vi "Main.vi"() -> ()   [LabVIEW 2018]
uses:
  TicTacToeControl.ctl
panel:
  out "array":string[](array[string])
  in  "stop":bool
  out "Display":string
  in  "Board":T1
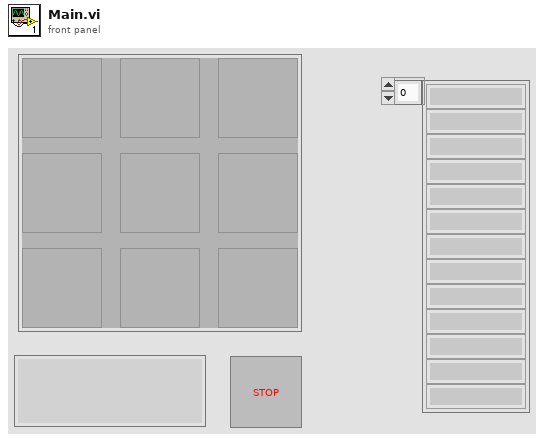
[diagram p1: front panel]
types:
  T1 = cluster{"OK Button":bool, "OK Button 2":bool, "OK Button 3":bool, "OK Button 4":bool, "OK Button 5":bool, "OK Button 6":bool, "OK Button 7":bool, "OK Button 8":bool, "OK Button 9":bool}
  T2 = typedef "TicTacToeControl.ctl" = enum16{"Initialize", "GetUserInput", "GetComputerMove", "SetControlValue", "Initialize Control References", "Wait for Event", "Quit", "Play Again ?", "Check result ?"}
  T3 = cluster{"Controls[]":refnum<vi>[], "selection index":i32, "user symbol":string, "computer symbol":string}
  T4 = typedef "gameStatus.ctl" = enum16{"player won", "computer won", "draw", "no result"}
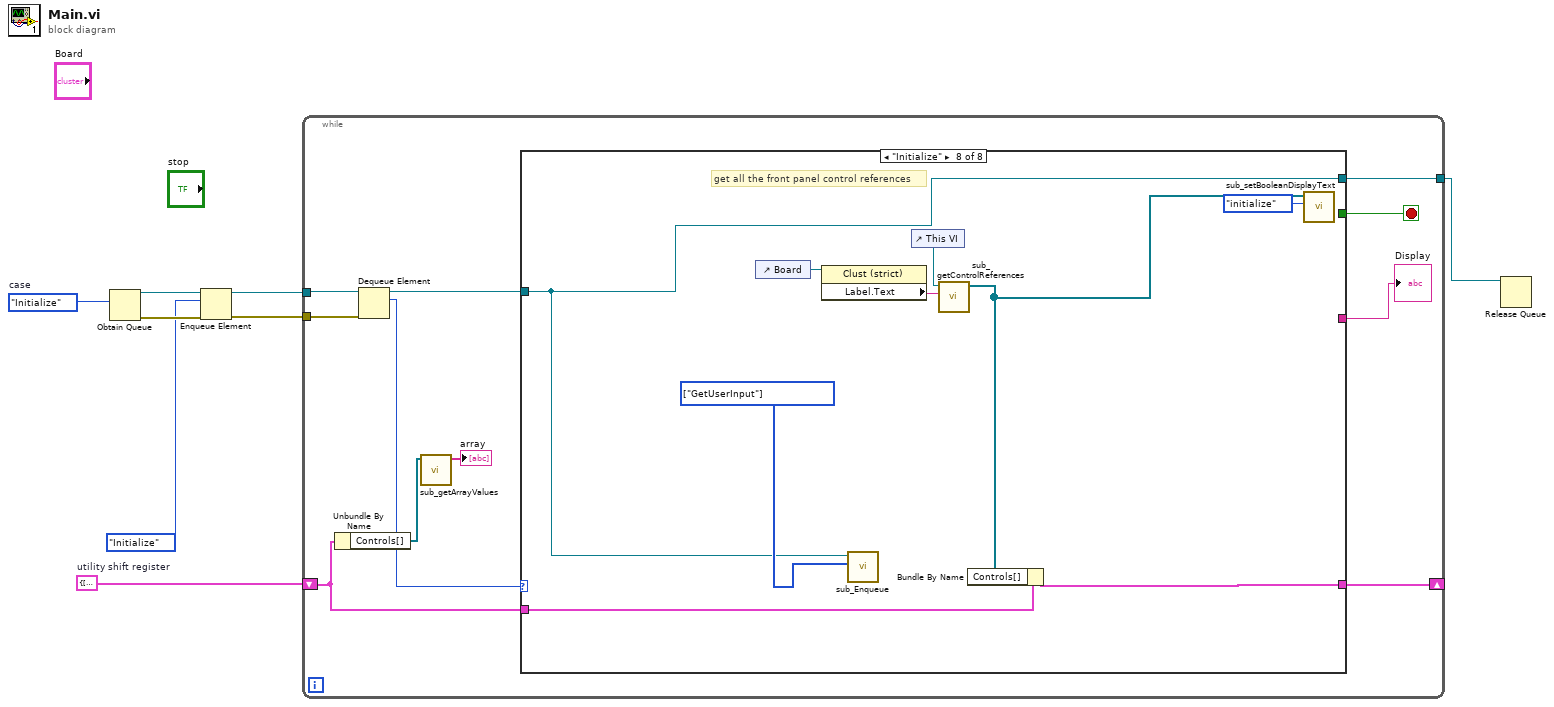
[diagram p0: block diagram]
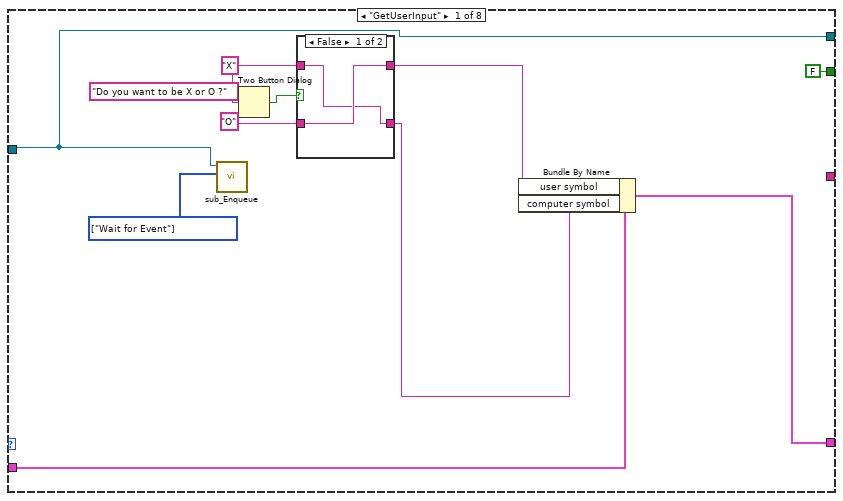
[diagram p2: hidden frame]
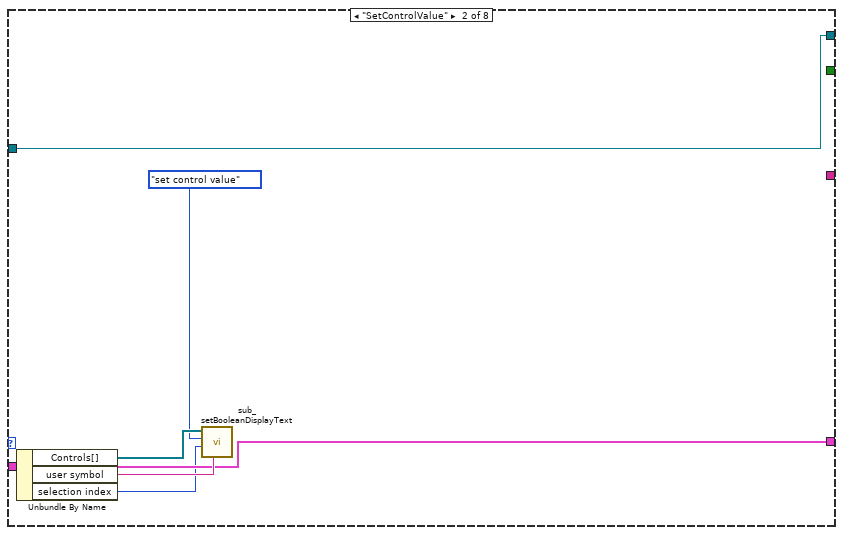
[diagram p4: hidden frame]
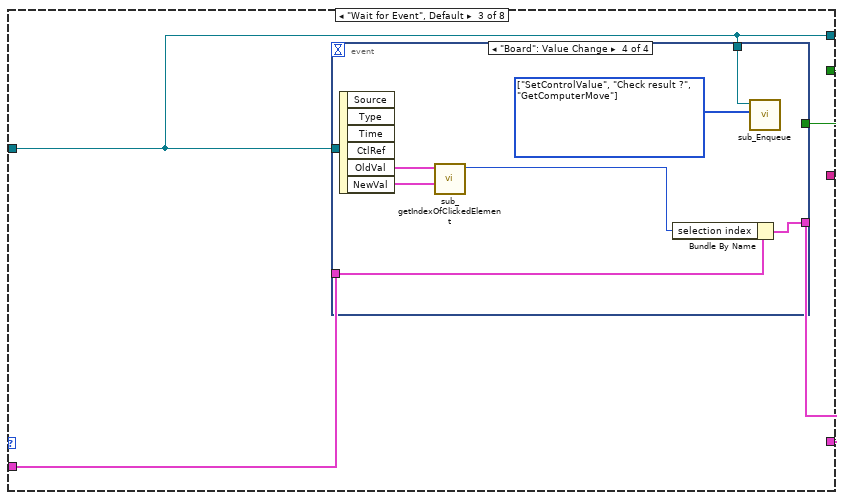
[diagram p5: hidden frame]
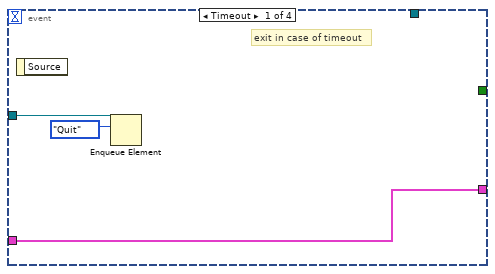
[diagram p6: hidden frame]
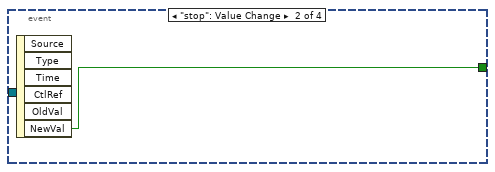
[diagram p7: hidden frame]
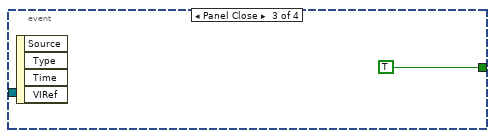
[diagram p8: hidden frame]
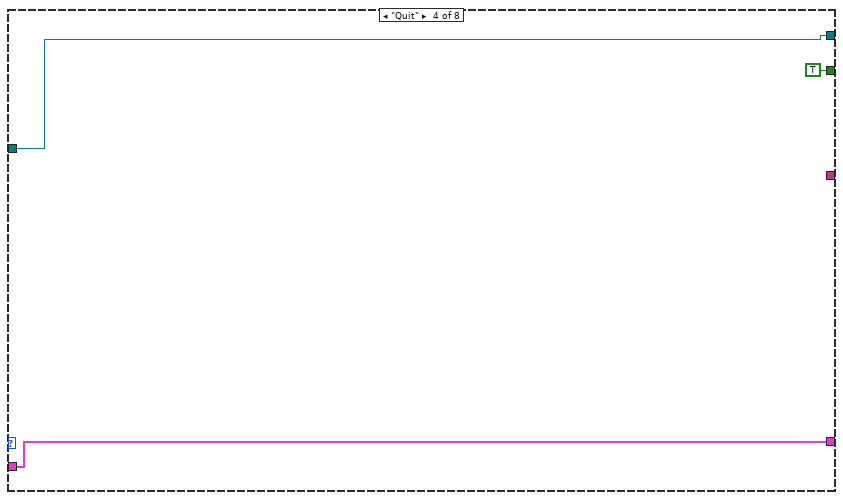
[diagram p9: hidden frame]
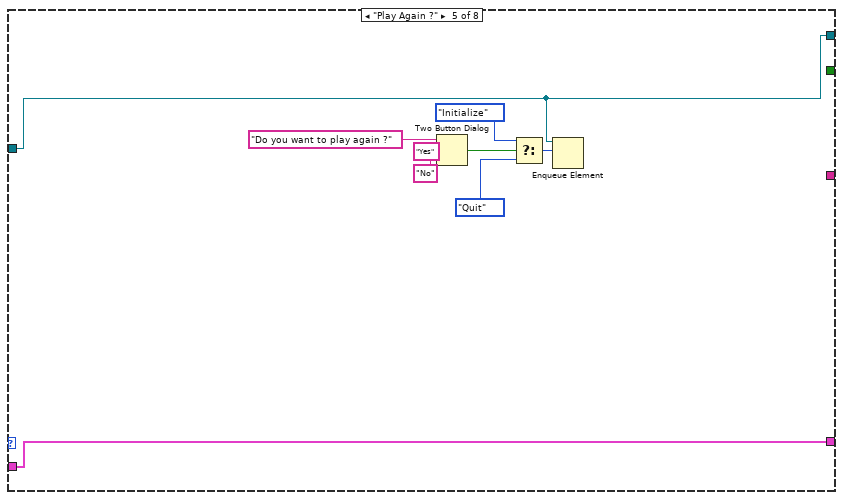
[diagram p10: hidden frame]
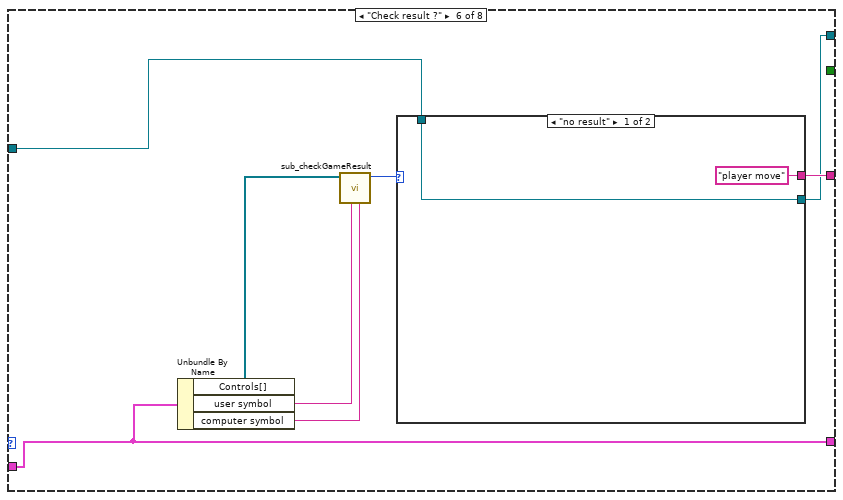
[diagram p11: hidden frame]
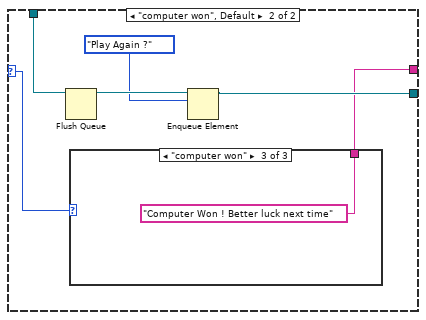
[diagram p12: hidden frame]
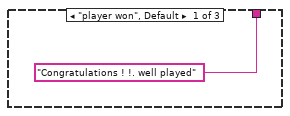
[diagram p13: hidden frame]
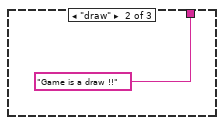
[diagram p14: hidden frame]
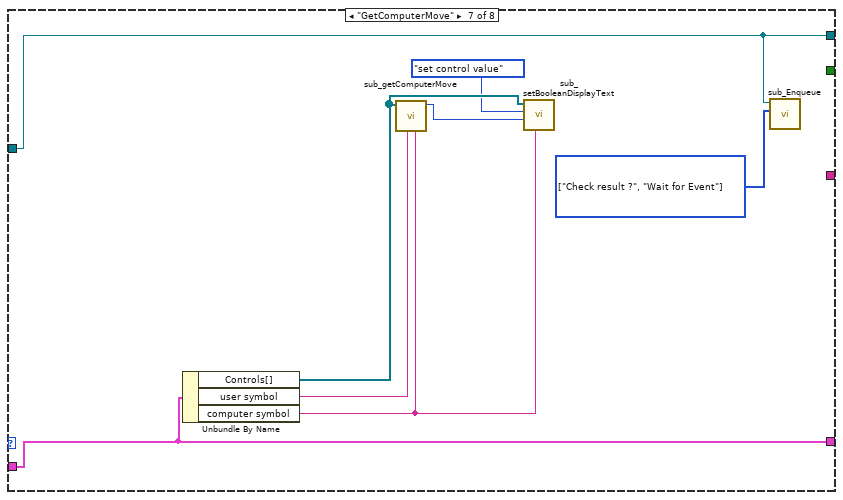
[diagram p15: hidden frame]
diagram:
  w8 = TicTacToeControl."Initialize"  # case
  w2 = T3 {"Controls[]"=[], "selection index"=0, "user symbol"="", "computer symbol"=""}  # utility shift register
  n1 = Obtain Queue(element data type=w8) -> (queue out=w7:refnum<queue>, error out=w6:errorcluster)  [unwired: 4 in, 1 out]
  n2 = Enqueue Element(queue=w7, element=TicTacToeControl."Initialize", error in (no error)=w6) -> (queue out=w4:refnum<queue>, error out=w3:errorcluster)  [unwired: 1 in, 1 out]
  n3 = while {
    shift-right: [w18] -> _
    shift-left: w2 -> [w11]
    tunnel: w4 -> [w17]
    tunnel: w3 -> [w16]
    tunnel: [w12] -> w1
    stop <- w19 stop-if-true
    n4 = Unbundle By Name(w11) -> ("Controls[]"=w10:refnum<vi>[])
    n5 = Dequeue Element(queue=w17, error in (no error)=w16) -> (queue out=w14:refnum<queue>, element=w15:T2)  [unwired: 1 in, 2 out]
    n6 = call "sub_getArrayValues.vi"("controls"=w10) -> ("array"=→"array":string[])  [unwired: 10 in]
    n7 = case shown="\"Initialize\"" w15 {
      tunnel: [FALSE _ w42 TRUE _ _ _ _] -> w19
      tunnel: w11 -> [w28 w39 w44 w58 w65 w76 w88 w101]
      tunnel: [w22 w39 w43 w58 w65 w76 w88 w100] -> w18
      tunnel: w14 -> [w20 w35 w41 w57 w60 w69 w90 w96]
      tunnel: [_ _ _ _ _ w75 _ _] -> w13
      tunnel: [w20 w35 w41 w57 w60 w70 w90 w96] -> w12
      frame "GetUserInput" {
        w21 = T2[] [enum."Wait for Event"] items=["Initialize", "GetUserInput", "GetComputerMove", "SetControlValue", "Initialize Control References", "Wait for Event", "Quit", "Play Again ?", "Check result ?"] ("commands")
        w24 = "O" ("F button name (\"Cancel\")")
        w26 = "X" ("T button name (\"OK\")")
        n8 = call "sub_Enqueue.vi"("commands"=w21, "queue"=w20) -> ()  [unwired: 10 in]
        n9 = Two Button Dialog(message="Do you want to be X or O ?", 1:w24, 2:w26) -> (T button?=w27:bool)
        n10 = case shown="False" w27 {
          tunnel: w26 -> [w31 w34]
          tunnel: [w32 w34] -> w25
          tunnel: w24 -> [w32 w33]
          tunnel: [w31 w33] -> w23
          frame False {
          }
          frame True {
          }
        }
        n11 = Bundle By Name(cluster=w28, "user symbol"=w25, "computer symbol"=w23) -> (w22:T3)
      }
      frame "SetControlValue" {
        n12 = Unbundle By Name(w39) -> ("Controls[]"=w38:refnum<vi>[], "user symbol"=w40:string, "selection index"=w36:i32)
        n13 = call "sub_setBooleanDisplayText.vi"("symbol"=w40, "selection index"=w36, "Enum"=enum16{"initialize", "set control value"}."set control value", "control references"=w38) -> ()  [unwired: 8 in]
      }
      frame "Wait for Event", Default {
        n14 = event shown="[3] \"Board\": Value Change" {
          selector: _ -> [_ _ _ _]
          dyn-events: _ -> [_ _ _ _]
          timeout: _ -> [_ _ _ _]
          tunnel: w44 -> [w47 _ _ w52]
          tunnel: [w47 _ _ w53] -> w43
          tunnel: [_ w48 TRUE _] -> w42
          tunnel: w41 -> [_ _ _ w51]
          tunnel: w41 -> [w46 _ _ _]
          event Timeout {
            # "exit in case of timeout"
            n15 = event-data() -> ()  [unwired: 1 in, 1 out]
            n16 = Enqueue Element(queue=w46, element=TicTacToeControl."Quit") -> ()  [unwired: 2 in, 3 out]
          }
          event "stop": Value Change {
            n17 = event-data() -> ("NewVal"=w48:bool)  [unwired: 1 in, 5 out]
          }
          event Panel Close {
            n18 = event-data() -> ()  [unwired: 1 in, 4 out]
          }
          event "Board": Value Change {
            w50 = T2[] [enum."SetControlValue", enum."Check result ?", enum."GetComputerMove"] items=["Initialize", "GetUserInput", "GetComputerMove", "SetControlValue", "Initialize Control References", "Wait for Event", "Quit", "Play Again ?", "Check result ?"] ("commands")
            n19 = event-data() -> ("OldVal"=w55:T1, "NewVal"=w56:T1)  [unwired: 1 in, 4 out]
            n20 = call "sub_getIndexOfClickedElement.vi"("NewVal"=w56, "OldVal"=w55) -> ("index of clicked element"=w54:i32)  [unwired: 9 in]
            n21 = Bundle By Name(cluster=w52, "selection index"=w54) -> (w53:T3)
            n22 = call "sub_Enqueue.vi"("commands"=w50, "queue"=w51) -> ()  [unwired: 10 in]
          }
        }
      }
      frame "Quit" {
      }
      frame "Play Again ?" {
        n23 = Two Button Dialog(message="Do you want to play again ?", 1:"No" ("F button name (\"Cancel\")"), 2:"Yes" ("T button name (\"OK\")")) -> (T button?=w64:bool)
        n24 = Select(t=TicTacToeControl."Initialize" ("element"), s=w64, f=TicTacToeControl."Quit") -> (s? t:f=w61:T2)
        n25 = Enqueue Element(queue=w60, element=w61) -> ()  [unwired: 2 in, 3 out]
      }
      frame "Check result ?" {
        n26 = Unbundle By Name(w76) -> ("Controls[]"=w74:refnum<vi>[], "user symbol"=w73:string, "computer symbol"=w72:string)
        n27 = call "sub_checkGameResult.vi"("computer symbol"=w72, "player symbol"=w73, "control references"=w74) -> ("game result"=w71:T4)  [unwired: 8 in]
        n28 = case shown="\"no result\"" w71 {
          selector: w71 -> [_ w80]
          tunnel: ["player move" w79] -> w75
          tunnel: [w77 w81] -> w70
          tunnel: w69 -> [w77 w84]
          frame "no result" {
          }
          frame "computer won", Default {
            n29 = Flush Queue(queue=w84) -> (queue out=w83:refnum<queue>)  [unwired: 1 in, 2 out]
            n30 = case shown="\"computer won\"" w80 {
              tunnel: ["Congratulations ! !. well played" "Game is a draw !!" "Computer Won ! Better luck next time"] -> w79
              frame "player won", Default {
              }
              frame "draw" {
              }
              frame "computer won" {
              }
            }
            n31 = Enqueue Element(queue=w83, element=TicTacToeControl."Play Again ?") -> (queue out=w81:refnum<queue>)  [unwired: 2 in, 2 out]
          }
        }
      }
      frame "GetComputerMove" {
        w89 = T2[] [enum."Check result ?", enum."Wait for Event"] items=["Initialize", "GetUserInput", "GetComputerMove", "SetControlValue", "Initialize Control References", "Wait for Event", "Quit", "Play Again ?", "Check result ?"] ("commands")
        n32 = Unbundle By Name(w88) -> ("Controls[]"=w94:refnum<vi>[], "user symbol"=w95:string, "computer symbol"=w91:string)
        n33 = call "sub_getComputerMove.vi"("player symbol"=w91, "computer symbol"=w95, "control references"=w94) -> ("computer move"=w92:i32)  [unwired: 8 in]
        n34 = call "sub_setBooleanDisplayText.vi"("symbol"=w91, "selection index"=w92, "Enum"=enum16{"initialize", "set control value"}."set control value", "control references"=w94) -> ()  [unwired: 8 in]
        n35 = call "sub_Enqueue.vi"("commands"=w89, "queue"=w90) -> ()  [unwired: 10 in]
      }
      frame "Initialize" {
        w97 = T2[] [enum."GetUserInput"] items=["Initialize", "GetUserInput", "GetComputerMove", "SetControlValue", "Initialize Control References", "Wait for Event", "Quit", "Play Again ?", "Check result ?"] ("commands")
        # "get all the front panel control references"
        n36 = control-ref of="Board"() -> (w103:refnum<vi>)
        n37 = property class="Clust (strict)"(reference=w103) -> ("Label.Text"=w104:string)  [unwired: 1 in, 2 out]
        n38 = call "sub_Enqueue.vi"("commands"=w97, "queue"=w96) -> ()  [unwired: 10 in]
        n39 = control-ref of="This VI"() -> (w102:refnum<vi>)
        n40 = call "sub_getControlReferences.vi"("board label"=w104, "VI in"=w102) -> ("Controls[]"=w99:refnum<vi>[])  [unwired: 8 in, 1 out]
        n41 = Bundle By Name(cluster=w101, "Controls[]"=w99) -> (w100:T3)
        n42 = call "sub_setBooleanDisplayText.vi"("Enum"=enum16{"initialize", "set control value"}."initialize", "control references"=w99) -> ()  [unwired: 10 in]
      }
    }
    "Display" <- w13
  }
  n43 = Release Queue(queue=w1) -> ()  [unwired: 2 in, 3 out]
